vi "2100_SP3T_SMU_Meas and Calculate Resitance_No Publish Data.vi"(7 "Current  Level":dbl=-0.01, 8 "error in (no error)":errorcluster, 10 "Pins":string[](array[string]), 11 "Semiconductor Module Context":T1) -> (0 "error Out":errorcluster, 1 "Individual_R_Meas":dbl[](array[numeric]), 2 "Mean_Meas_Current":dbl[](array[numeric]), 3 "Semiconductor Module Context Out":T1, 4 "Mean_Meas_Voltage":dbl[](array[numeric]))   [LabVIEW 2013]
uses:
  <vilib>/NI_TestStand_SemiconductorModule/NI_TestStand_Semiconductor_Module.lvlibp/PinMap/General/SemiconductorModuleContext.ctl
  <vilib>/Analysis/baseanly.llb/Mean (DBL).vi
  <vilib>/NI_TestStand_SemiconductorModule/NI_TestStand_Semiconductor_Module.lvlibp/PinMap/DC Power/PinsToNIDCPowerSessions.vi
  <vilib>/NI_TestStand_SemiconductorModule/NI_TestStand_Semiconductor_Module.lvlibp
  <vilib>/Analysis/NI_AALBase.lvlib
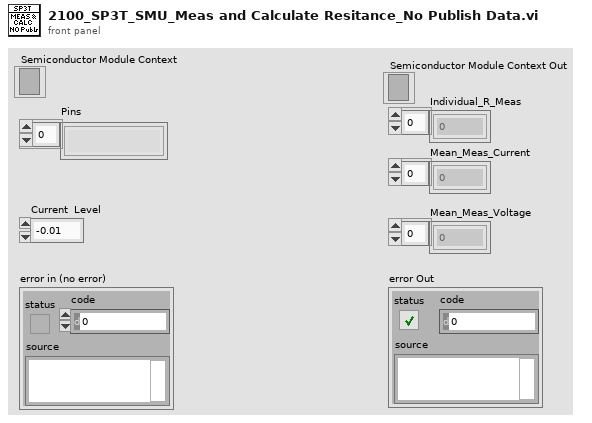
[diagram p1: front panel]
types:
  T1 = typedef "NI_TestStand_Semiconductor_Module.lvlibp/SemiconductorModuleContext.ctl" = refnum<k7>
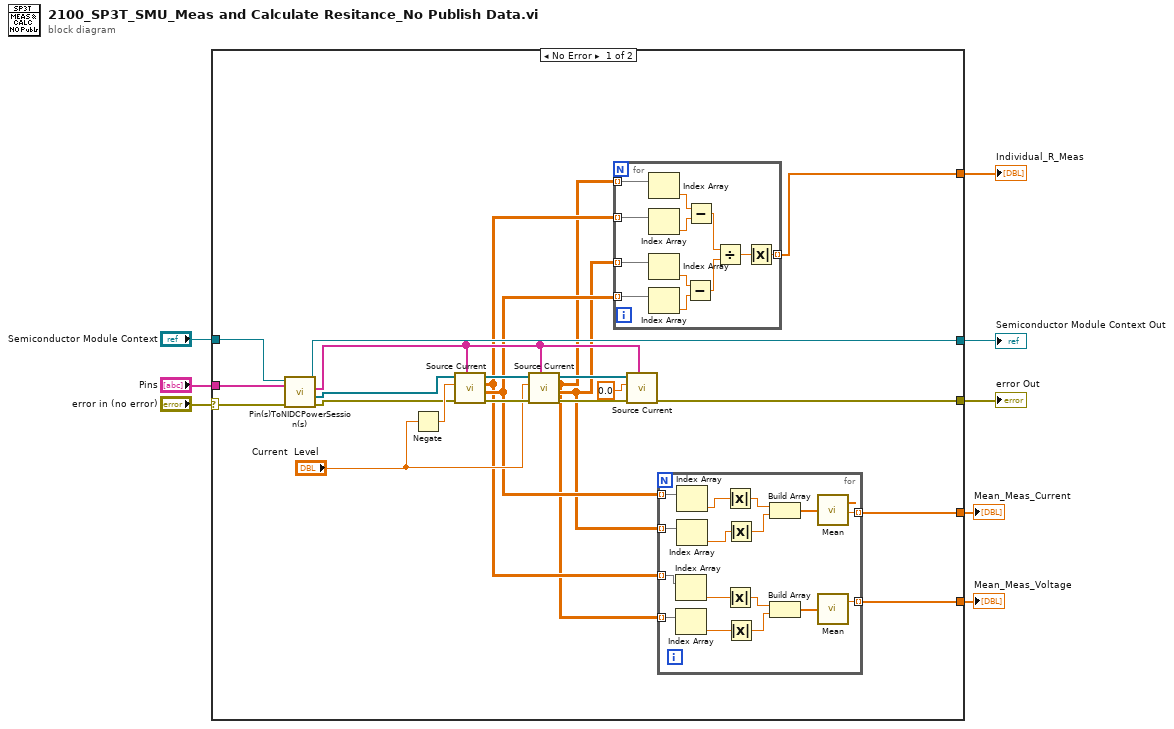
[diagram p0: block diagram]
diagram:
  n1 = case shown="No Error" "error in (no error)" {
    selector: "error in (no error)" -> [w30 w60]
    tunnel: "Semiconductor Module Context" -> [w28 w59]
    tunnel: "Pins" -> [w29 _]
    tunnel: [w18 w60] -> w5
    tunnel: [w17 w59] -> w4
    tunnel: [w15 _] -> w3
    tunnel: [w12 _] -> w2
    tunnel: [w9 _] -> w1
    frame No Error {
      n2 = call-poly <vilib>:"Pin(s)ToNIDCPowerSession(s).vi"("error in (no error)"=w30, "Pins"=w29, "Semiconductor Module Context"=w28) -> ("error out"=w20:errorcluster, "Instrument Sessions"=w19:refnum<k15>[], "Channel Lists"=w16:string[], "Semiconductor Module Context Out"=w17:T1)  [unwired: 4 in, 1 out]
      n3 = Negate(x="Current  Level") -> (-x=w26:dbl)
      n4 = call "Source Current.vi"("Channel Lists"=w16, "error in (no error)"=w20, "current level"=w26, "Instrument Sessions In"=w19) -> ("error out"=w25:errorcluster, "current measurements"=w14:dbl[][], "voltage measurements"=w11:dbl[][], "Instrument Sessions Out"=w24:refnum<k15>[])  [unwired: 4 in]
      n5 = call "Source Current.vi"("Channel Lists"=w16, "error in (no error)"=w25, "current level"="Current  Level", "Instrument Sessions In"=w24) -> ("error out"=w23:errorcluster, "current measurements"=w13:dbl[][], "voltage measurements"=w10:dbl[][], "Instrument Sessions Out"=w27:refnum<k15>[])  [unwired: 4 in]
      n6 = for {
        tunnel: w10 -> [w51] mode=indexing
        tunnel: w13 -> [w58] mode=indexing
        tunnel: [w56] -> w15 mode=indexing
        tunnel: w14 -> [w55] mode=indexing
        tunnel: w11 -> [w48] mode=indexing
        n7 = Index Array(array=w51) -> (element=w50:dbl)  [unwired: 1 in]
        n8 = Index Array(array=w48) -> (element=w49:dbl)  [unwired: 1 in]
        n9 = Index Array(array=w58) -> (element=w52:dbl)  [unwired: 1 in]
        n10 = Index Array(array=w55) -> (element=w54:dbl)  [unwired: 1 in]
        n11 = Subtract(x=w52, y=w54) -> (x-y=w53:dbl)
        n12 = Subtract(x=w50, y=w49) -> (x-y=w47:dbl)
        n13 = Divide(x=w47, y=w53) -> (x/y=w57:dbl)
        n14 = Absolute Value(x=w57) -> (abs(x)=w56:dbl)
      }
      n15 = call "Source Current.vi"("Channel Lists"=w16, "error in (no error)"=w23, "current level"=0.0, "Instrument Sessions In"=w27) -> ("error out"=w18:errorcluster)  [unwired: 4 in, 3 out]
      n16 = for {
        tunnel: w14 -> [w46] mode=indexing
        tunnel: w13 -> [w45] mode=indexing
        tunnel: [w31] -> w12 mode=indexing
        tunnel: w11 -> [w39] mode=indexing
        tunnel: w10 -> [w38] mode=indexing
        tunnel: [w37] -> w9 mode=indexing
        n17 = Index Array(array=w39) -> (element=w43:dbl)  [unwired: 1 in]
        n18 = Index Array(array=w38) -> (element=w44:dbl)  [unwired: 1 in]
        n19 = Index Array(array=w46) -> (element=w33:dbl)  [unwired: 1 in]
        n20 = Index Array(array=w45) -> (element=w32:dbl)  [unwired: 1 in]
        n21 = Absolute Value(x=w33) -> (abs(x)=w35:dbl)
        n22 = Absolute Value(x=w43) -> (abs(x)=w41:dbl)
        n23 = Absolute Value(x=w32) -> (abs(x)=w36:dbl)
        n24 = Absolute Value(x=w44) -> (abs(x)=w42:dbl)
        n25 = Build Array(w35, w36) -> (w34:dbl[])
        n26 = Build Array(w41, w42) -> (w40:dbl[])
        n27 = call-poly <vilib>:"Mean.vi"("X"=w34) -> ("mean"=w31:dbl)  [unwired: 1 out]
        n28 = call-poly <vilib>:"Mean.vi"("X"=w40) -> ("mean"=w37:dbl)  [unwired: 1 out]
      }
    }
    frame Error {
    }
  }
  "error Out" <- w5
  "Semiconductor Module Context Out" <- w4
  "Individual_R_Meas" <- w3
  "Mean_Meas_Current" <- w2
  "Mean_Meas_Voltage" <- w1
